vi "Task3.vi"() -> ()   [LabVIEW 2017]
panel:
  in  "stop":bool
  out "Numeric":dbl
  in  "Button":bool[](array[boolean])
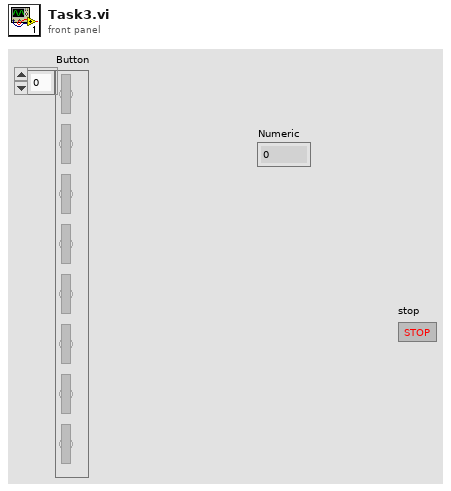
[diagram p1: front panel]
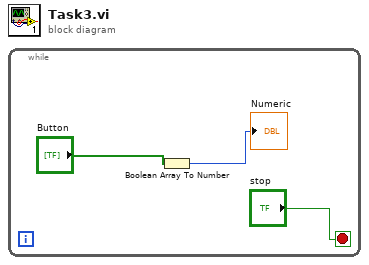
[diagram p0: block diagram]
diagram:
  n1 = while {
    stop <- "stop" stop-if-true
    n2 = Boolean Array To Number(Boolean array="Button") -> (number=→"Numeric":u32)
  }
